vi "Main 17052018.vi"() -> ()   [LabVIEW 2016]
uses:
  Control/Settings.ctl
  Control/port config.ctl
  <vilib>/LabVIEW Interface for Arduino/Type Defs/Board Type.ctl
  Queue Message Handler/Message Queue.lvlib
  <vilib>/LabVIEW Interface for Arduino/LabVIEW Interface for Arduino.lvlib
panel:
  out "Filterd":dbl[](graph)
  out "Saving":bool
  out "Settings out":T1={"Port"={"Port Name"="", "Board Type"=enum."Uno", "Baud Rate"=115200}, "Sample Rate (HZ)"=100, "Samples to Read"=50, "Input Pin"=0, "File path saved"=path ""}
  out "Spectrum":dbl[](graph)
  out "Raw data":dbl[](graph)
  in  "End":bool
  in  "Record Button":bool
  in  "Start":bool
  in  "Settings port":bool
  out "error out":errorcluster={"status"=FALSE, "code"=1073676294, "source"="VISA Read in LabVIEW Interface for Arduino.lvlib:Send Receive.vi->LabVIEW Interface for Arduino.lvlib:Continuous Acquisition Off.vi->Main.vi"}
  in  "stop logging":bool
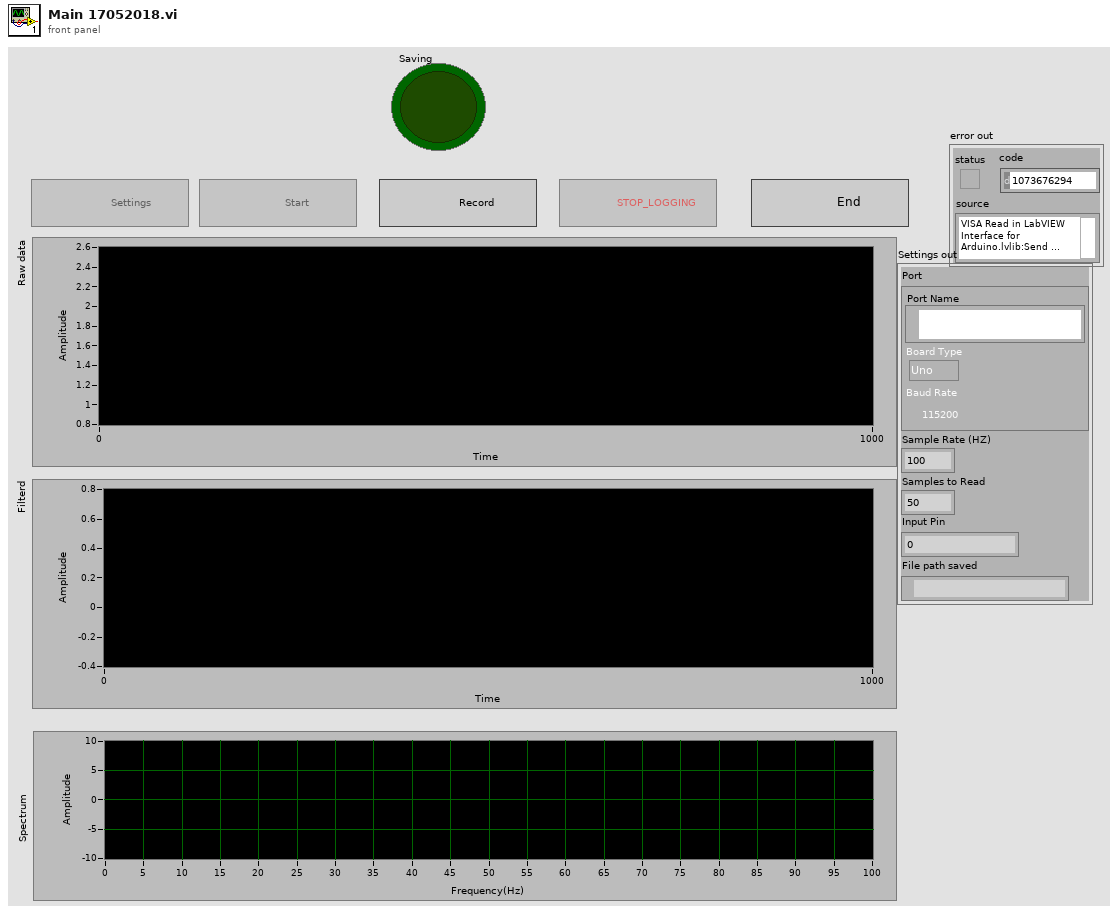
[diagram p1: front panel]
types:
  T1 = typedef "Settings.ctl" = cluster{"Port":T2, "Sample Rate (HZ)":u16, "Samples to Read":u16, "Input Pin":u8, "File path saved":path}
  T2 = typedef "port config.ctl" = cluster{"Port Name":refnum<visa-resource-name>, "Board Type":T3, "Baud Rate":u32}
  T3 = typedef "LabVIEW Interface for Arduino.lvlib/Board Type.ctl" = enum16{"Uno", "Dimuelanove w/Atmega 328", "Mega 2560"}
  T4 = enum8{"Enabled", "Disabled", "Disabled and Grayed Out"}
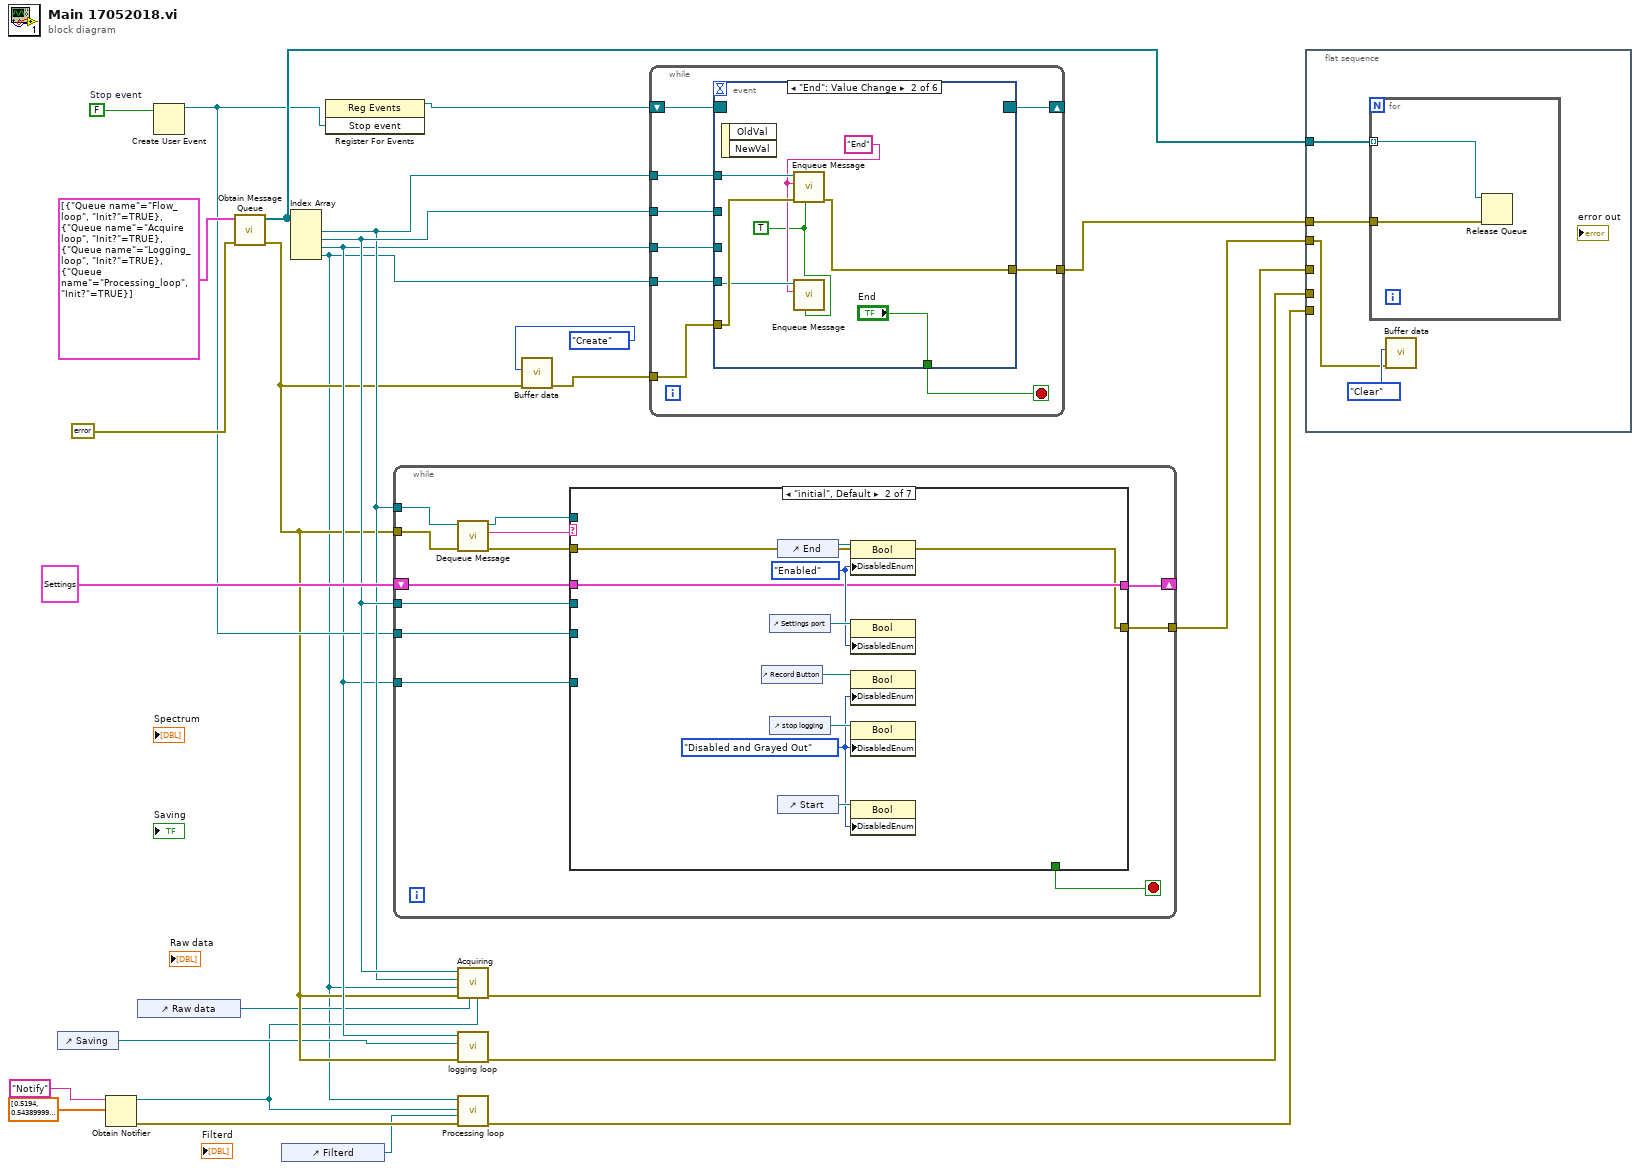
[diagram p0: block diagram]
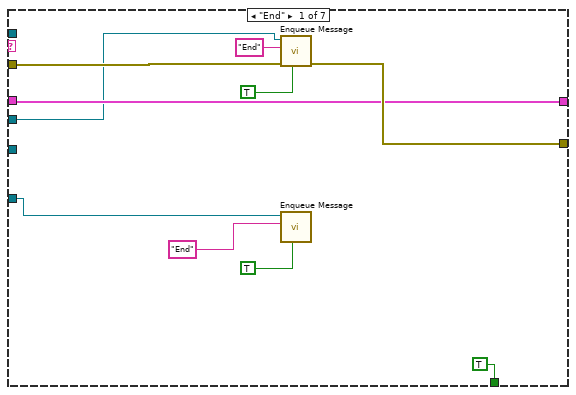
[diagram p2: hidden frame]
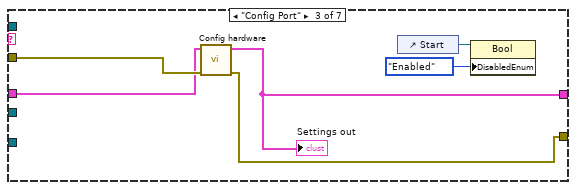
[diagram p3: hidden frame]
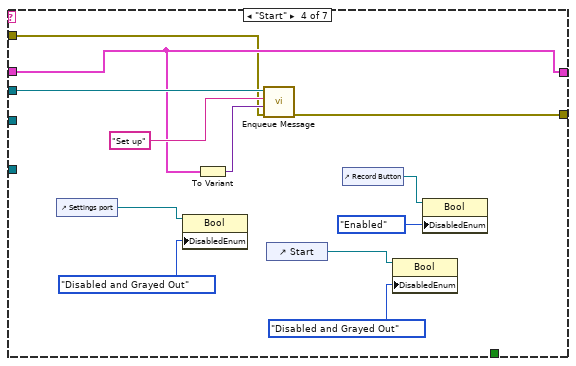
[diagram p4: hidden frame]
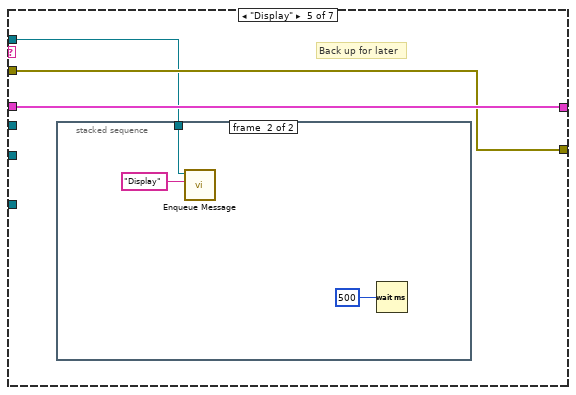
[diagram p5: hidden frame]
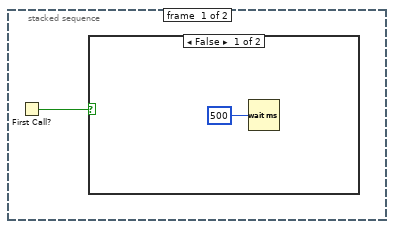
[diagram p6: hidden frame]
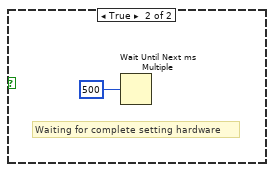
[diagram p7: hidden frame]
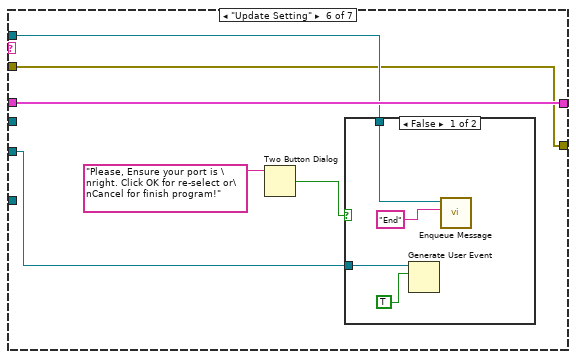
[diagram p8: hidden frame]
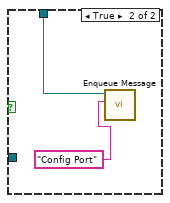
[diagram p9: hidden frame]
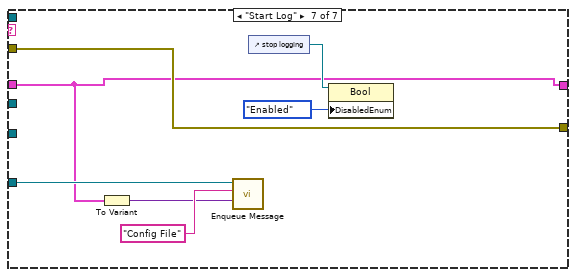
[diagram p10: hidden frame]
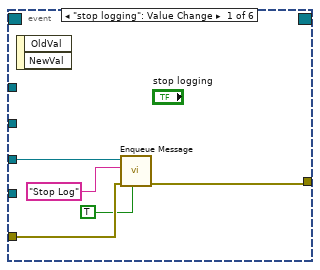
[diagram p11: hidden frame]
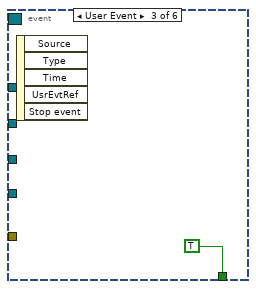
[diagram p12: hidden frame]
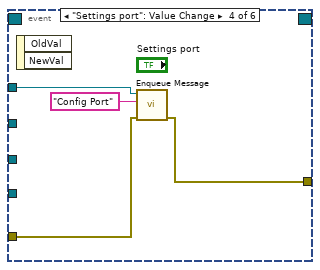
[diagram p13: hidden frame]
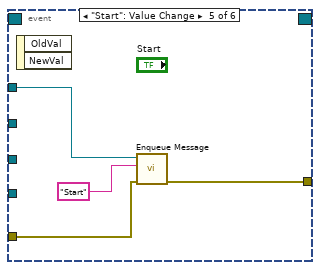
[diagram p14: hidden frame]
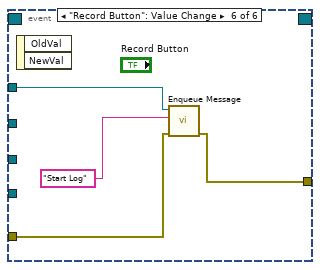
[diagram p15: hidden frame]
diagram:
  w15 = FALSE  # Stop event
  n1 = control-ref of="Saving"() -> (w9:refnum<vi>)
  n2 = Obtain Notifier(name (unnamed)="Notify", notification data type=dbl[] [0.5194, 0.5438999999999999, 0.5095999999999999, 0.539, 0.49979999999999997, 0.5341, 0.49, 0.5341, 0.4851, 0.5292, 0.48019999999999996, 0.5292, 0.4753, 0.5341, 0.4753, 0.5341, 0.4753, 0.539, 0.4753, 0.539, 0.4753, 0.5438999999999999, 0.4704, 0.5488, 0.4704, 0.5488, 0.4753, 0.5488, 0.4753, 0.5488, 0.48019999999999996, 0.5488, 0.48019999999999996, 0.5488, 0.48019999999999996, 0.5438999999999999, 0.4851, 0.5438999999999999, 0.49, 0.5438999999999999, 0.4949, 0.539, 0.4949, 0.539, 0.49979999999999997, 0.5341, 0.49979999999999997, 0.5341, 0.5047, 0.5341] ("Raw data")) -> (notifier out=w5:refnum<notifier>, error out=w3:errorcluster)  [unwired: 2 in, 1 out]
  n3 = control-ref of="Raw data"() -> (w8:refnum<vi>)
  n4 = Create User Event(user event datatype=w15) -> (user event=w14:refnum<user-event>)  [unwired: 1 in, 1 out]
  n5 = call "Obtain Message Queue.vi"("error in (no error)"=errorcluster {"status"=FALSE, "code"=0, "source"=""}, "Queue config"=cluster{"Queue name":string, "Init?":bool}[] [{"Queue name"="Flow_loop", "Init?"=TRUE}, {"Queue name"="Acquire loop", "Init?"=TRUE}, {"Queue name"="Logging_loop", "Init?"=TRUE}, {"Queue name"="Processing_loop", "Init?"=TRUE}]) -> ("error out"=w11:errorcluster, "Queue out"=w24:refnum<queue>[])  [unwired: 8 in]
  n6 = control-ref of="Filterd"() -> (w1:refnum<vi>)
  n7 = Index Array(array=w24) -> (element #1=w16:refnum<queue>, element #2=w21:refnum<queue>, element #3=w12:refnum<queue>, element #4=w4:refnum<queue>)  [unwired: 4 in]
  n8 = register-events(w14) -> (reference out=w13:refnum<event-registration>)  [unwired: 2 in, 1 out]
  n9 = while {
    tunnel: w16 -> [w37]
    tunnel: w11 -> [w36]
    shift-right: [w33] -> _
    shift-left: T1 {"Port"={"Port Name"="", "Board Type"=enum."Uno", "Baud Rate"=115200}, "Sample Rate (HZ)"=100, "Samples to Read"=50, "Input Pin"=0, "File path saved"=path ""} ("Settings out") -> [w32]
    tunnel: w21 -> [w31]
    tunnel: [w30] -> w20
    tunnel: w14 -> [w28]
    tunnel: w12 -> [w27]
    stop <- w34 stop-if-true
    n10 = call "Dequeue Message.vi"("error in (no error)"=w36, "Message Queue"=w37) -> ("error out"=w35:errorcluster, "Message"=w38:string, "dup Message Queue"=w29:refnum<queue>)  [unwired: 6 in, 1 out]
    n11 = case shown="\"initial\", Default" w38 {
      tunnel: w35 -> [w45 w49 w61 w69 w77 w86 w101]
      tunnel: [TRUE _ _ _ _ _ _] -> w34
      tunnel: [w46 w50 w60 w70 w78 w90 w97] -> w33
      tunnel: w32 -> [w46 w50 w59 w70 w78 w90 w97]
      tunnel: w31 -> [w42 _ _ w73 _ _ _]
      tunnel: [w47 w49 w58 w68 w77 w86 w101] -> w30
      tunnel: w29 -> [_ _ _ _ w76 w87 _]
      tunnel: w28 -> [_ _ _ _ _ w85 _]
      tunnel: w27 -> [w41 _ _ _ _ _ w100]
      frame "End" {
        n12 = call "Enqueue Message.vi"("Priority Message? (F)"=TRUE, "error in (no error)"=w45, "Message"="End", "Message Queue"=w42) -> ("error out"=w47:errorcluster)  [unwired: 6 in, 1 out]
        n13 = call "Enqueue Message.vi"("Priority Message? (F)"=TRUE, "Message"="End", "Message Queue"=w41) -> ()  [unwired: 7 in, 2 out]
      }
      frame "initial", Default {
        w52 = T4."Disabled and Grayed Out" ("Disabled")
        w51 = T4."Enabled" ("Disabled")
        n14 = control-ref of="Record Button"() -> (w55:refnum<vi>)
        n15 = control-ref of="Settings port"() -> (w56:refnum<vi>)
        n16 = control-ref of="stop logging"() -> (w54:refnum<vi>)
        n17 = control-ref of="End"() -> (w53:refnum<vi>)
        n18 = control-ref of="Start"() -> (w57:refnum<vi>)
        n19 = property class="Bool"(reference=w53, "DisabledEnum"=w51) -> ()  [unwired: 1 in, 2 out]
        n20 = property class="Bool"(reference=w56, "DisabledEnum"=w51) -> ()  [unwired: 1 in, 2 out]
        n21 = property class="Bool"(reference=w55, "DisabledEnum"=w52) -> ()  [unwired: 1 in, 2 out]
        n22 = property class="Bool"(reference=w54, "DisabledEnum"=w52) -> ()  [unwired: 1 in, 2 out]
        n23 = property class="Bool"(reference=w57, "DisabledEnum"=w52) -> ()  [unwired: 1 in, 2 out]
      }
      frame "Config Port" {
        n24 = call "Config hardware.vi"("error in"=w61, "Settings"=w59) -> ("error out"=w58:errorcluster, "Settings out"=w60:T1)  [unwired: 8 in]
        "Settings out" <- w60
        n25 = control-ref of="Start"() -> (w63:refnum<vi>)
        n26 = property class="Bool"(reference=w63, "DisabledEnum"=T4."Enabled" ("Disabled")) -> ()  [unwired: 1 in, 2 out]
      }
      frame "Start" {
        n27 = control-ref of="Settings port"() -> (w67:refnum<vi>)
        n28 = property class="Bool"(reference=w67, "DisabledEnum"=T4."Disabled and Grayed Out" ("Disabled")) -> ()  [unwired: 1 in, 2 out]
        n29 = To Variant(anything=w70) -> (Variant=w71:variant)
        n30 = call "Enqueue Message.vi"("error in (no error)"=w69, "Message Data"=w71, "Message"="Set up", "Message Queue"=w73) -> ("error out"=w68:errorcluster)  [unwired: 6 in, 1 out]
        n31 = control-ref of="Start"() -> (w64:refnum<vi>)
        n32 = control-ref of="Record Button"() -> (w74:refnum<vi>)
        n33 = property class="Bool"(reference=w64, "DisabledEnum"=T4."Disabled and Grayed Out" ("Disabled")) -> ()  [unwired: 1 in, 2 out]
        n34 = property class="Bool"(reference=w74, "DisabledEnum"=T4."Enabled" ("Disabled")) -> ()  [unwired: 1 in, 2 out]
      }
      frame "Display" {
        # "Back up for later"
        n35 = stacked-sequence {
          tunnel: w76 -> [_ w84]
          frame #0 {
            n36 = First Call?() -> (First Call?: T/F=w79:bool)
            n37 = case shown="False" w79 {
              frame False {
                n38 = Wait (ms)(milliseconds to wait=u32 500) -> ()  [unwired: 1 out]
              }
              frame True {
                # "Waiting for complete setting hardware"
                n39 = Wait Until Next ms Multiple(millisecond multiple=u32 500) -> ()  [unwired: 1 out]
              }
            }
          }
          frame #1 {
            n40 = call "Enqueue Message.vi"("Message"="Display", "Message Queue"=w84) -> ()  [unwired: 8 in, 2 out]
            n41 = Wait (ms)(milliseconds to wait=u32 500) -> ()  [unwired: 1 out]
          }
        }
      }
      frame "Update Setting" {
        n42 = Two Button Dialog(message="Please, Ensure your port is \nright. Click OK for re-select or\nCancel for finish program!") -> (T button?=w88:bool)  [unwired: 2 in]
        n43 = case shown="False" w88 {
          tunnel: w87 -> [w94 w96]
          tunnel: w85 -> [w92 _]
          frame False {
            n44 = Generate User Event(user event=w92, event data cluster=TRUE ("Stop event")) -> ()  [unwired: 2 in, 2 out]
            n45 = call "Enqueue Message.vi"("Message"="End", "Message Queue"=w94) -> ()  [unwired: 8 in, 2 out]
          }
          frame True {
            n46 = call "Enqueue Message.vi"("Message"="Config Port", "Message Queue"=w96) -> ()  [unwired: 8 in, 2 out]
          }
        }
      }
      frame "Start Log" {
        n47 = To Variant(anything=w97) -> (Variant=w98:variant)
        n48 = call "Enqueue Message.vi"("Message Data"=w98, "Message"="Config File", "Message Queue"=w100) -> ()  [unwired: 7 in, 2 out]
        n49 = control-ref of="stop logging"() -> (w102:refnum<vi>)
        n50 = property class="Bool"(reference=w102, "DisabledEnum"=T4."Enabled" ("Disabled")) -> ()  [unwired: 1 in, 2 out]
      }
    }
  }
  n51 = call "Acquiring.vi"("Notify"=w5, "GrphChrt Refnum"=w8, "error in"=w11, "Processing Queue"=w4, "Flow Queue"=w16, "Acquire Queue"=w21) -> ("error out"=w19:errorcluster)  [unwired: 5 in]
  n52 = call "logging loop.vi"("error in"=w11, "Saving"=w9, "Log queue"=w12) -> ("error out"=w10:errorcluster)  [unwired: 8 in]
  n53 = call "Processing loop.vi"("error in"=w3, "Signal"=w1, "Notify"=w5, "Processing Queue"=w4) -> ("error out"=w2:errorcluster)  [unwired: 7 in]
  n54 = call "Buffer data.vi"("Error in"=w11, "Command"=enum16{"Create", "Enqueue", "Dequeue", "Clear"}."Create") -> ("error out"=w18:errorcluster)  [unwired: 8 in, 1 out]
  n55 = while {
    tunnel: w16 -> [w111]
    tunnel: w21 -> [w110]
    tunnel: w12 -> [w109]
    tunnel: w18 -> [w108]
    tunnel: [w107] -> w23
    shift-right: [w105] -> _
    shift-left: w13 -> [w106]
    tunnel: w4 -> [w104]
    stop <- w112 stop-if-true
    n56 = event shown="[1] \"End\": Value Change" {
      selector: w106 -> [_ _ _ _ _ _]
      dyn-events: [_ _ _ _ _ _] -> w105
      timeout: _ -> [_ _ _ _ _ _]
      tunnel: [_ "End" TRUE _ _ _] -> w112
      tunnel: w111 -> [_ w123 _ w129 w130 w137]
      tunnel: w110 -> [_ _ _ _ _ _]
      tunnel: w109 -> [w114 _ _ _ _ _]
      tunnel: w108 -> [w116 w122 _ w127 w132 w135]
      tunnel: [w115 w121 _ w126 w131 w134] -> w107
      tunnel: w104 -> [_ w120 _ _ _ _]
      event "stop logging": Value Change {
        n57 = event-data() -> ()  [unwired: 1 in, 2 out]
        n58 = call "Enqueue Message.vi"("Priority Message? (F)"=TRUE, "error in (no error)"=w116, "Message"="Stop Log", "Message Queue"=w114) -> ("error out"=w115:errorcluster)  [unwired: 6 in, 1 out]
      }
      event "End": Value Change {
        w118 = TRUE ("Priority Message? (F)")
        w119 = "End" ("Message")
        n59 = event-data() -> ()  [unwired: 1 in, 2 out]
        n60 = call "Enqueue Message.vi"("Priority Message? (F)"=w118, "error in (no error)"=w122, "Message"=w119, "Message Queue"=w123) -> ("error out"=w121:errorcluster)  [unwired: 6 in, 1 out]
        n61 = call "Enqueue Message.vi"("Priority Message? (F)"=w118, "Message"=w119, "Message Queue"=w120) -> ()  [unwired: 7 in, 2 out]
      }
      event User Event {
        n62 = event-data() -> ()  [unwired: 1 in, 5 out]
      }
      event "Settings port": Value Change {
        n63 = event-data() -> ()  [unwired: 1 in, 2 out]
        n64 = call "Enqueue Message.vi"("error in (no error)"=w127, "Message"="Config Port", "Message Queue"=w129) -> ("error out"=w126:errorcluster)  [unwired: 7 in, 1 out]
      }
      event "Start": Value Change {
        n65 = event-data() -> ()  [unwired: 1 in, 2 out]
        n66 = call "Enqueue Message.vi"("error in (no error)"=w132, "Message"="Start", "Message Queue"=w130) -> ("error out"=w131:errorcluster)  [unwired: 7 in, 1 out]
      }
      event "Record Button": Value Change {
        n67 = event-data() -> ()  [unwired: 1 in, 2 out]
        n68 = call "Enqueue Message.vi"("error in (no error)"=w135, "Message"="Start Log", "Message Queue"=w137) -> ("error out"=w134:errorcluster)  [unwired: 7 in, 1 out]
      }
    }
  }
  n69 = flat-sequence {
    tunnel: w24 -> [w140]
    tunnel: w23 -> [w141]
    tunnel: w20 -> [w138]
    tunnel: w19 -> [_]
    tunnel: w10 -> [_]
    tunnel: w2 -> [_]
    frame #0 {
      n70 = for {
        tunnel: w141 -> [w143]
        tunnel: w140 -> [w142] mode=indexing
        n71 = Release Queue(queue=w142, error in (no error)=w143) -> ()  [unwired: 1 in, 3 out]
      }
      n72 = call "Buffer data.vi"("Error in"=w138, "Command"=enum16{"Create", "Enqueue", "Dequeue", "Clear"}."Clear") -> ()  [unwired: 8 in, 2 out]
    }
  }
